vi "Test Simple String.vi"() -> ()   [LabVIEW 2013]
uses:
  PopupMenu Plugin/JKI SM Helper.llb/JKI SM Helper Source.ctl
  <vilib>/Utility/miscctls.llb/LVPositionTypeDef.ctl
panel:
  out "Menu Items To Add":T1(array[cluster])
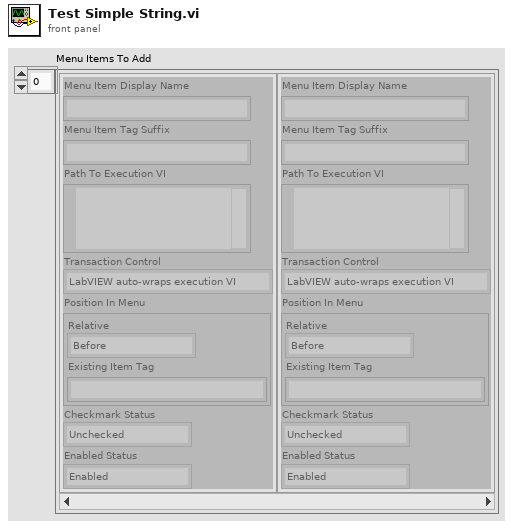
[diagram p1: front panel]
types:
  T1 = cluster{"Menu Item Display Name":string, "Menu Item Tag Suffix":string, "Path To Execution VI":path, "Transaction Control":enum8{"LabVIEW auto-wraps execution VI", "Execution VI will define if needed"}, "Position In Menu":cluster{"Relative":enum8{"Before", "Instead of", "After", "Into Submenu"}, "Existing Item Tag":string}, "Checkmark Status":enum8{"Unchecked", "Checked"}, "Enabled Status":enum8{"Enabled", "Disabled"}}[]
  T2 = typedef "LVPositionTypeDef.ctl" = cluster{"Left":i32, "Top":i32}
  T3 = typedef "JKI SM Helper Source.ctl" = cluster{"Case Structure":refnum<vi>[], "Event Structure":refnum<vi>[], "While Loop":refnum<vi>[], "String Constant":refnum<vi>[], "Named Bundler":refnum<vi>[], "Named Unbundler":refnum<vi>[], "InPlaceClusterNode":refnum<vi>[]}
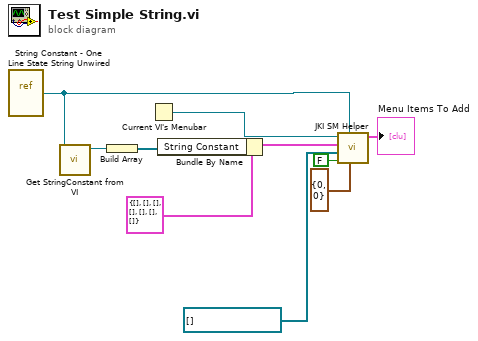
[diagram p0: block diagram]
diagram:
  n1 = vi-ref "String Constant - One Line State String Unwired.vi"() -> (w4:refnum<vi>)
  n2 = call "Get StringConstant from VI.vi"("VI in"=w4) -> ("StringConstant out"=w9:refnum<vi>)  [unwired: 9 in, 1 out]
  n3 = Build Array(w9) -> (w8:refnum<vi>[])
  n4 = Current VI's Menubar() -> (w2:refnum<k9>)
  n5 = Bundle By Name(cluster=T3 {"Case Structure"=[], "Event Structure"=[], "While Loop"=[], "String Constant"=[], "Named Bundler"=[], "Named Unbundler"=[], "InPlaceClusterNode"=[]} ("Affected Items"), "String Constant"=w8) -> (w7:T3)
  n6 = call "JKI SM Helper.vi"("Mouse Position"=T2 {"Left"=0, "Top"=0}, "User VI Ref"=w4, "Is Multi-select?"=FALSE, "Remaining Items"=refnum<vi>[] [], "Affected Items"=w7, "Menu Refnum"=w2) -> ("Menu Items To Add"=→"Menu Items To Add":T1)  [unwired: 5 in]
